vi "SLM Ctrl Make Mode Name Array.vi"() -> ()   [LabVIEW 2018]
uses:
  SLM Control TypeDefs/SLM Ctrl Mode Names.ctl
panel:
  out "JSON string":string
  in  "ModeNamesArray":T1
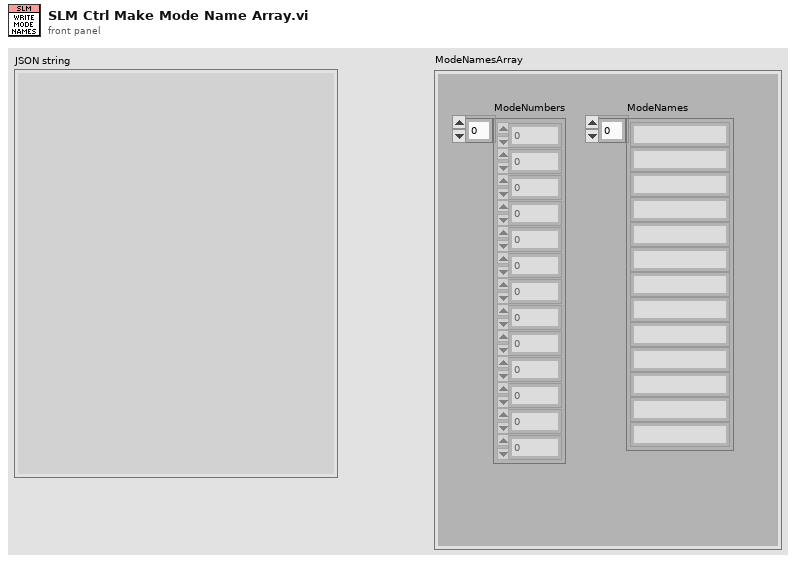
[diagram p1: front panel]
types:
  T1 = typedef "SLM Ctrl Mode Names.ctl" = cluster{"ModeNumbers":u8[], "ModeNames":string[]}
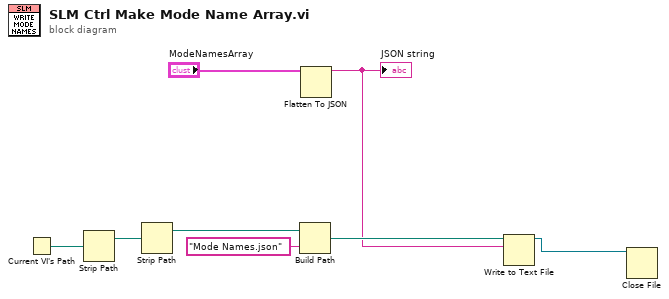
[diagram p0: block diagram]
diagram:
  n1 = Current VI's Path() -> (path=w7:path)
  n2 = Strip Path(path=w7) -> (stripped path=w6:path)  [unwired: 1 out]
  n3 = Strip Path(path=w6) -> (stripped path=w5:path)  [unwired: 1 out]
  n4 = Build Path(base path=w5, name or relative path="Mode Names.json") -> (appended path=w3:path)
  n5 = Flatten To JSON(anything="ModeNamesArray") -> (JSON string=w1:string)  [unwired: 2 in, 1 out]
  "JSON string" <- w1
  n6 = Write to Text File(file (use dialog)=w3, text=w1) -> (refnum out=w2:refnum<file>)  [unwired: 2 in, 2 out]
  n7 = Close File(refnum=w2) -> ()  [unwired: 1 in, 2 out]
